vi "DDS.vi"(1 "Device":string, 2 "In":variant, 3 "Mode":u32(ring) items=["Open", "Close", "Begin", "End", "Get", "Set"]) -> (0 "Out":variant)   [LabVIEW 2014]
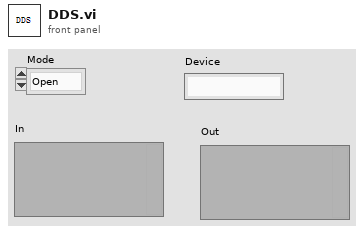
[diagram p1: front panel]
types:
  T1 = enum16{"Standard", "Buffered", "CRLF", "Immediate"}
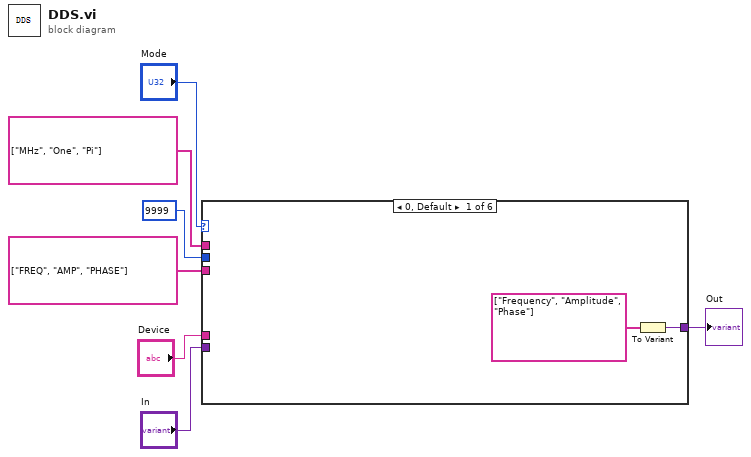
[diagram p0: block diagram]
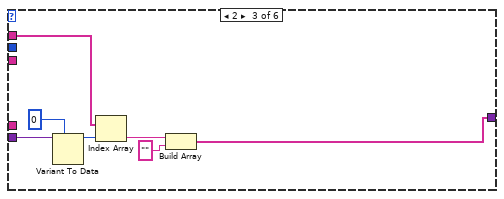
[diagram p3: hidden frame]
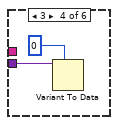
[diagram p4: hidden frame]
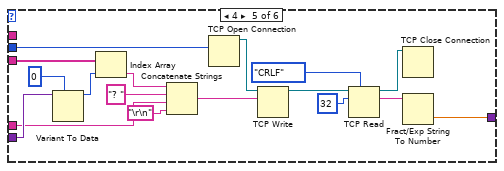
[diagram p5: hidden frame]
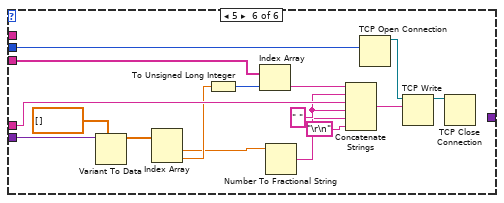
[diagram p6: hidden frame]
diagram:
  n1 = case shown="0, Default" "Mode" {
    tunnel: "In" -> [_ _ w16 w17 w35 w51]
    tunnel: [w8 _ w10 _ w24 _] -> w6
    tunnel: string[] ["MHz", "One", "Pi"] ("Strings []") -> [_ _ w13 _ _ _]
    tunnel: u16 9999 ("remote port or service name") -> [_ _ _ _ w25 w42]
    tunnel: "Device" -> [_ _ _ _ w22 w46]
    tunnel: string[] ["FREQ", "AMP", "PHASE"] ("Strings []") -> [_ _ _ _ w21 w47]
    frame 0, Default {
      n2 = To Variant(anything=string[] ["Frequency", "Amplitude", "Phase"] ("Strings []")) -> (Variant=w8:variant)
    }
    frame 1 {
    }
    frame 2 {
      n3 = Variant To Data(type=0, Variant=w16) -> (data=w12:i32)  [unwired: 1 in, 1 out]
      n4 = Index Array(array=w13, index=w12) -> (element=w11:string)
      n5 = Build Array(w11, "") -> (w10:string[])
    }
    frame 3 {
      n6 = Variant To Data(type=0, Variant=w17) -> ()  [unwired: 1 in, 2 out]
    }
    frame 4 {
      n7 = Variant To Data(type=u32 0, Variant=w35) -> (data=w19:u32)  [unwired: 1 in, 1 out]
      n8 = Index Array(array=w21, index=w19) -> (element=w28:string)
      n9 = Concatenate Strings(w28, "? " ("string"), w22, "\r\n") -> (w26:string)
      n10 = TCP Open Connection(remote port or service name=w25) -> (connection ID=w29:refnum<k5>)  [unwired: 4 in, 1 out]
      n11 = TCP Write(connection ID=w29, data in=w26) -> (connection ID out=w30:refnum<k5>)  [unwired: 2 in, 2 out]
      n12 = TCP Read(connection ID=w30, bytes to read=32, 7:T1."CRLF" ("mode (standard)")) -> (connection ID out=w32:refnum<k5>, data out=w31:string)  [unwired: 2 in, 1 out]
      n13 = TCP Close Connection(connection ID=w32) -> ()  [unwired: 2 in, 2 out]
      n14 = Fract/Exp String To Number(string=w31) -> (number=w24:dbl)  [unwired: 3 in, 1 out]
    }
    frame 5 {
      w44 = " " ("string")
      n15 = Variant To Data(type=dbl[] [] ("appended array"), Variant=w51) -> (data=w39:dbl[])  [unwired: 1 in, 1 out]
      n16 = Index Array(array=w39) -> (element #1=w36:dbl, element #2=w38:dbl)  [unwired: 2 in]
      n17 = To Unsigned Long Integer(number=w38) -> (unsigned 32bit integer=w37:u32)
      n18 = Index Array(array=w47, index=w37) -> (element=w49:string)
      n19 = Number To Fractional String(number=w36) -> (F-format string=w41:string)  [unwired: 3 in]
      n20 = Concatenate Strings(w49, w44, w46, w44, w41, "\r\n") -> (w48:string)
      n21 = TCP Open Connection(remote port or service name=w42) -> (connection ID=w50:refnum<k5>)  [unwired: 4 in, 1 out]
      n22 = TCP Write(connection ID=w50, data in=w48) -> (connection ID out=w43:refnum<k5>)  [unwired: 2 in, 2 out]
      n23 = TCP Close Connection(connection ID=w43) -> ()  [unwired: 2 in, 2 out]
    }
  }
  "Out" <- w6
